vi "Main.vi"   [LabVIEW 2021]
uses:
  Dev Actor/Dev Actor/Dev Actor.lvclass
  C:/git/jettl/temp/Dev Actor/Dev Actor/Dev Actor.lvclass
  C:/git/jettl/temp/Msgs/Pop Up/Pop Up/Pop Up.lvclass
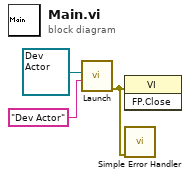
[diagram p0: block diagram]
diagram:
  n1 = call <vilib>:"Launch.vi"("Alias"="Dev Actor", "Actor"=refnum<class "Dev Actor.lvclass"> refnum ("Process.lvlib:Process.lvclass")) -> ("error out"=w1:errorcluster)  [unwired: 9 in]
  n2 = invoke class="VI" method="FP.Close"(error in=w1) -> ()  [unwired: 2 in, 3 out]
  n3 = call <vilib>:"Simple Error Handler.vi"("error in (no error)"=w1) -> ()  [unwired: 4 in, 5 out]
